vi "PlotMag.vi"(8 "error in (no error)":errorcluster, 11 "AllData In":T1 {"FlukeData"."DataAnalysisArray"."TimeStamp" format="%^<%.3X\n%x>T"; "FlukeData"."ModelDataArray"."FREQUENCY" format="%#_6f"; "FlukeData"."ModelDataArray"."TimeStamp" format="%^<%.3X\n%x>T"; "FlukeData"."PMUDataArray"."FREQUENCY" format="%#_6f"; "FlukeData"."PMUDataArray"."TimeStamp" format="%^<%.3X\n%x>T"; "NISTData"."DataAnlysisArray"."TimeStamp" format="%^<%.3X\n%x>T"; "NISTData"."DUTDataArray"."Time Stamp" format="%^<%.3X\n%x>T"; "NISTData"."NIDataArray"."Time Stamp" format="%^<%.3X\n%x>T"}) -> (0 "error out":errorcluster, 1 "NistPlot":cluster{"X":dbl, "Y":dbl}[](array[cluster]), 2 "FlukePlot":cluster{"X":dbl, "Y":dbl}[](array[cluster]))   [LabVIEW 2014]
uses:
  typedefs/Alldata.ctl
  typedefs/NISTData.ctl
  typedefs/NIDataArray.ctl
  typedefs/NIData.ctl
  typedefs/PhasorRectangular.ctl
  typedefs/DUTData.ctl
  typedefs/NICalcAnalysis.ctl
  typedefs/CalcPhasorError.ctl
  typedefs/PlotDataArrays.ctl
  typedefs/PmuRawDataCluster.ctl
  typedefs/CalcAnalysis.ctl
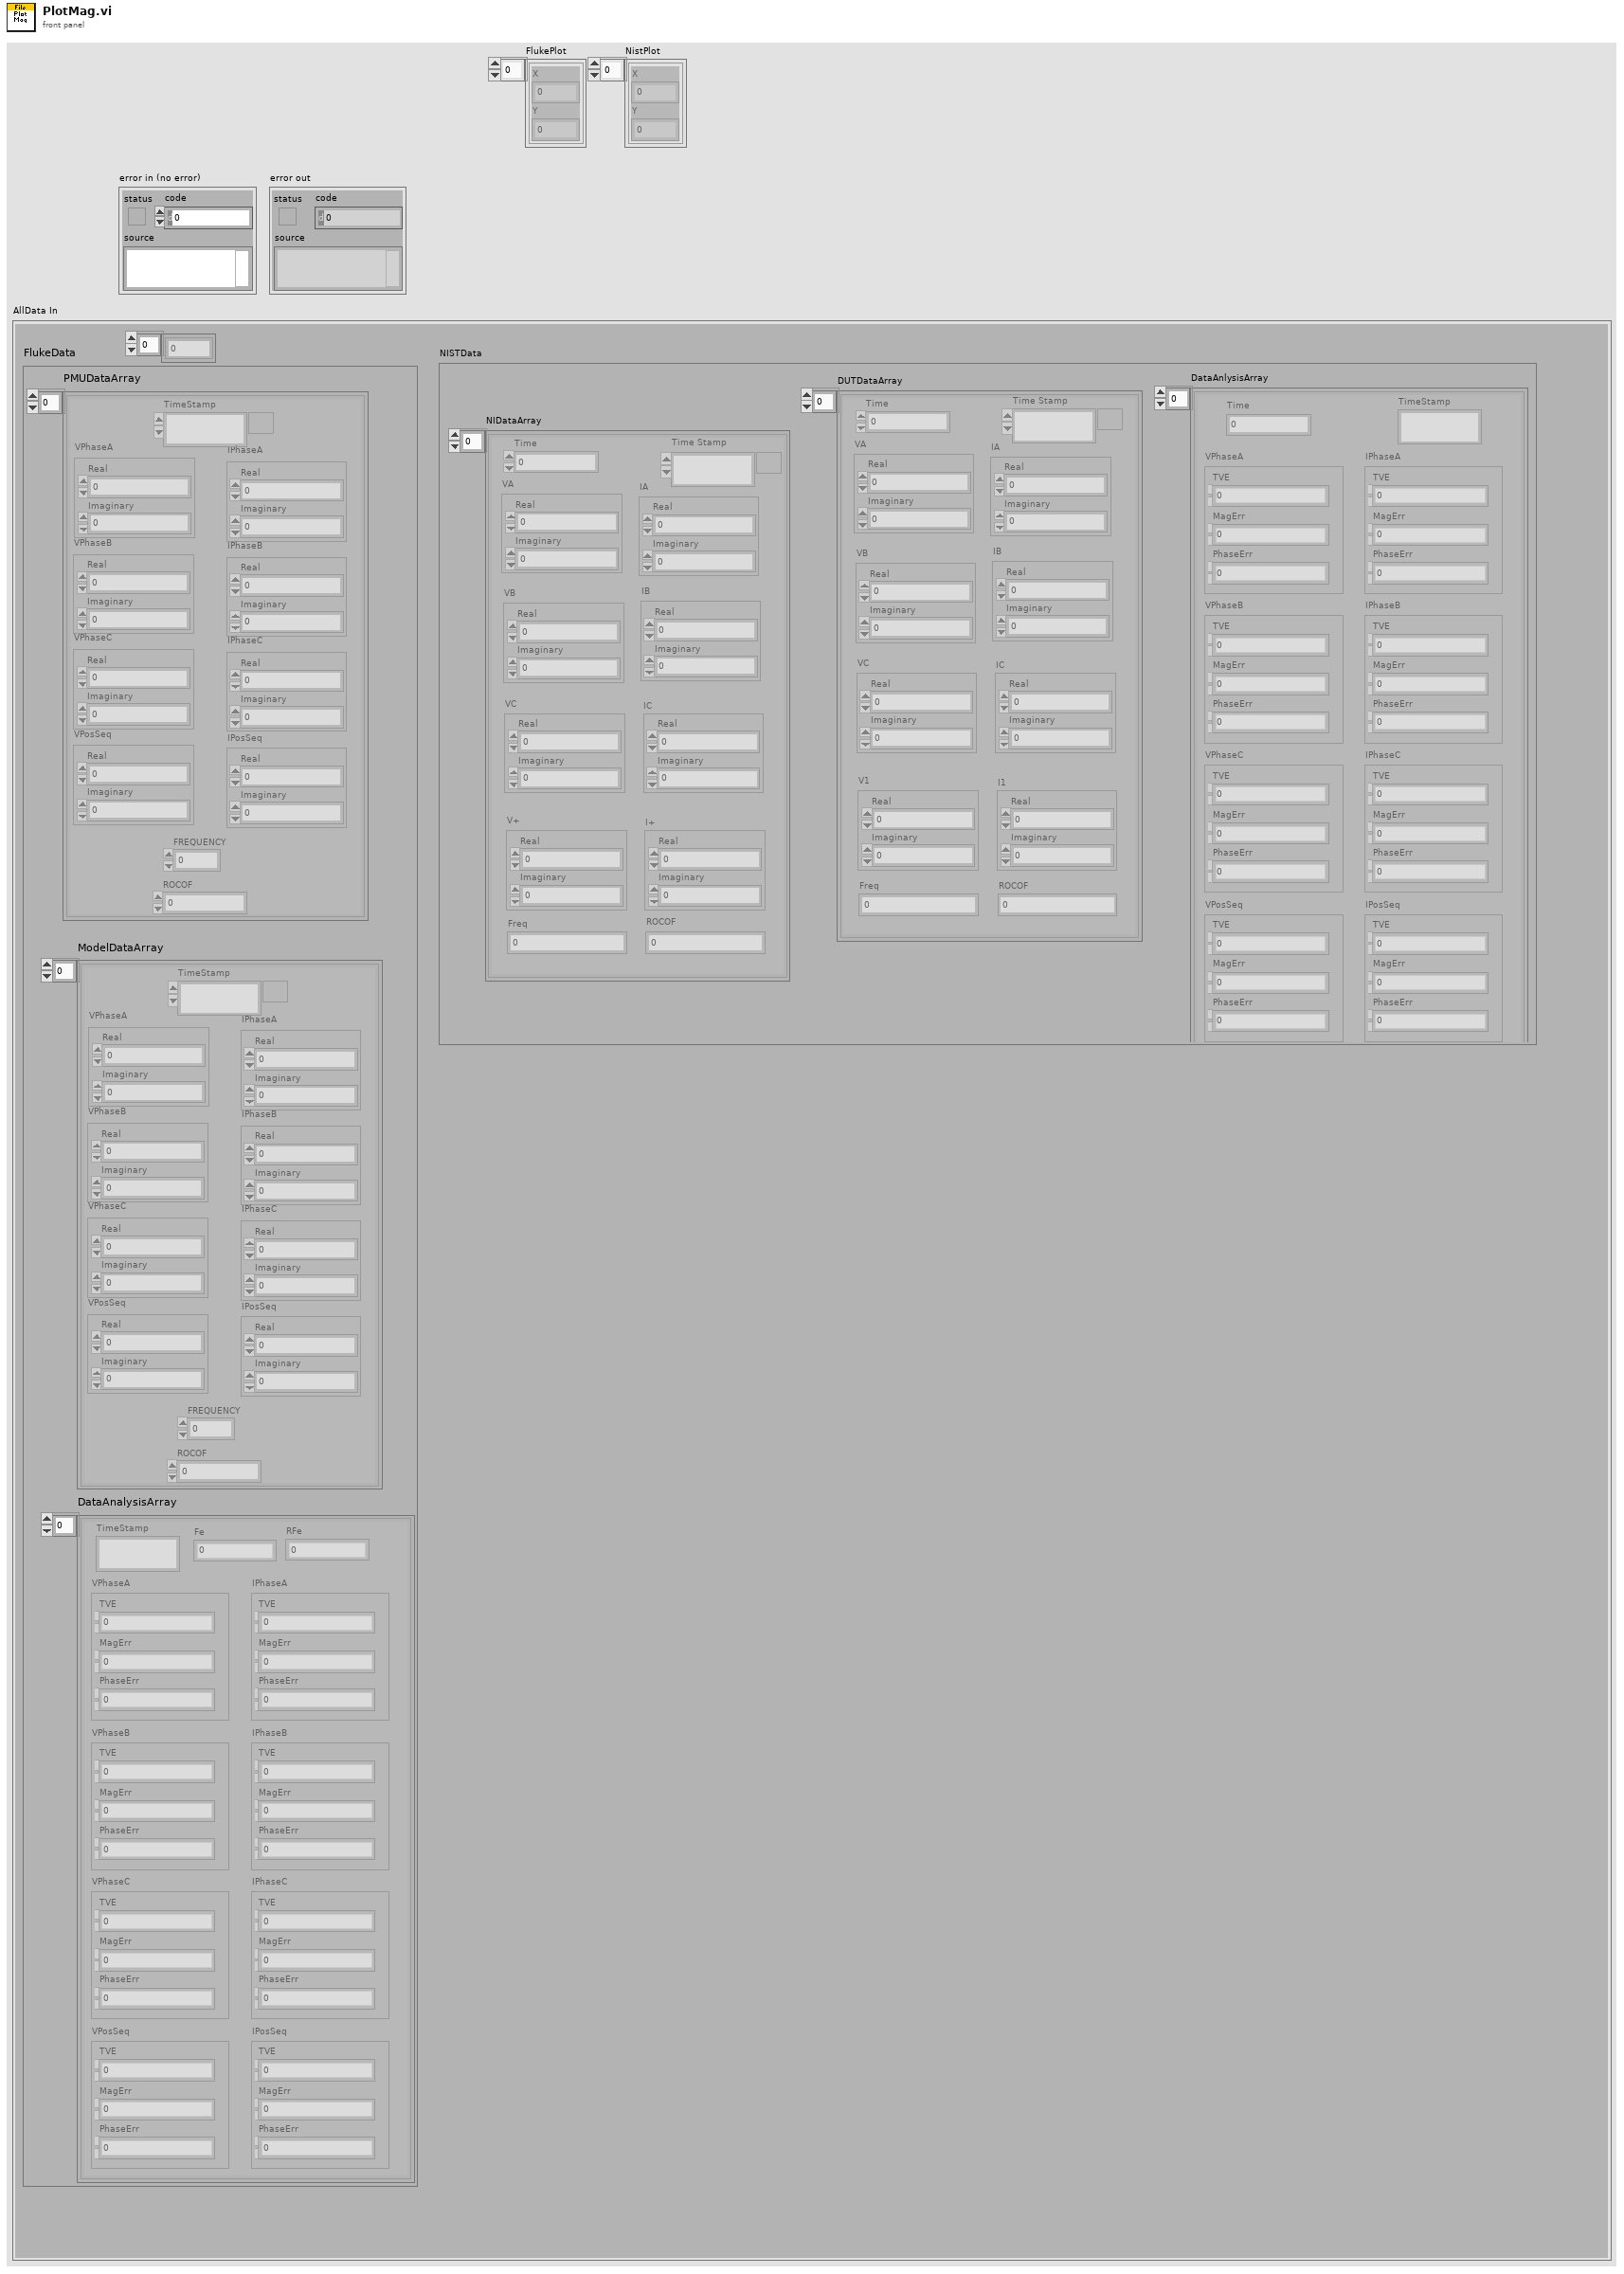
[diagram p1: front panel]
types:
  T1 = typedef "Alldata.ctl" = cluster{"NISTData":T2, "FlukeData":T9, "Params":dbl[]}
  T2 = typedef "NISTData.ctl" = cluster{"NIDataArray":T3, "DUTDataArray":T6[], "DataAnlysisArray":T7[]}
  T3 = typedef "NIDataArray.ctl" = T4[]
  T4 = typedef "NIData.ctl" = cluster{"Time":dbl, "VA":T5, "VB":T5, "VC":T5, "V+":T5, "IA":T5, "IB":T5, "IC":T5, "I+":T5, "Freq":dbl, "ROCOF":dbl, "Time Stamp":timestamp}
  T5 = typedef "PhasorRectangular.ctl" = cluster{"Real":dbl, "Imaginary":dbl}
  T6 = typedef "DUTData.ctl" = cluster{"Time":dbl, "VA":T5, "VB":T5, "VC":T5, "V1":T5, "IA":T5, "IB":T5, "IC":T5, "I1":T5, "Freq":dbl, "ROCOF":dbl, "Time Stamp":timestamp}
  T7 = typedef "NICalcAnalysis.ctl" = cluster{"Time":dbl, "VPhaseA":T8, "IPhaseA":T8, "VPhaseB":T8, "IPhaseB":T8, "VPhaseC":T8, "IPhaseC":T8, "VPosSeq":T8, "IPosSeq":T8, "Fe":dbl, "RFe":dbl, "TimeStamp":timestamp}
  T8 = typedef "CalcPhasorError.ctl" = cluster{"TVE":dbl, "MagErr":dbl, "PhaseErr":dbl}
  T9 = typedef "PlotDataArrays.ctl" = cluster{"PMUDataArray":T10[], "ModelDataArray":T10[], "DataAnalysisArray":T11[]}
  T10 = typedef "PmuRawDataCluster.ctl" = cluster{"TimeStamp":timestamp, "VPhaseA":T5, "VPhaseB":T5, "VPhaseC":T5, "VPosSeq":T5, "IPhaseA":T5, "IPhaseB":T5, "IPhaseC":T5, "IPosSeq":T5, "FREQUENCY":dbl, "ROCOF":sgl}
  T11 = typedef "CalcAnalysis.ctl" = cluster{"TimeStamp":timestamp, "VPhaseA":T8, "VPhaseB":T8, "VPhaseC":T8, "VPosSeq":T8, "IPhaseA":T8, "IPhaseB":T8, "IPhaseC":T8, "IPosSeq":T8, "Fe":dbl, "RFe":dbl}
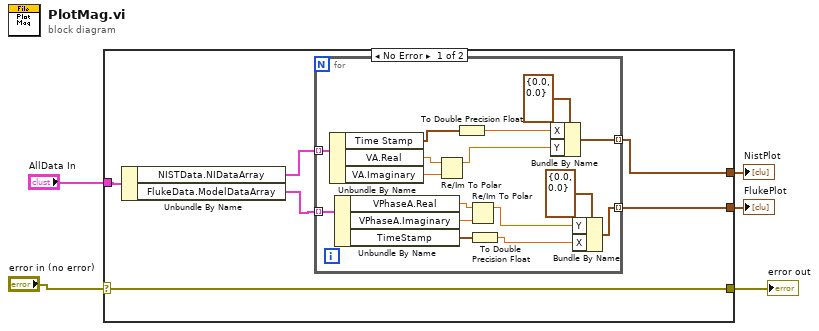
[diagram p0: block diagram]
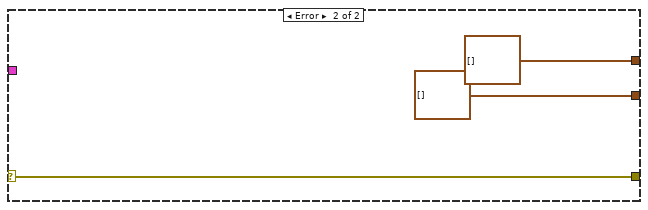
[diagram p2: hidden frame]
diagram:
  n1 = case shown="No Error" "error in (no error)" {
    selector: "error in (no error)" -> [w7 w30]
    tunnel: [w7 w30] -> w4
    tunnel: "AllData In" -> [w11 _]
    tunnel: [w6 cluster{"X":dbl, "Y":dbl}[] []] -> w1
    tunnel: [w8 cluster{"X":dbl, "Y":dbl}[] []] -> w2
    frame No Error {
      n2 = Unbundle By Name(w11) -> ("NISTData.NIDataArray"=w10:T3, "FlukeData.ModelDataArray"=w9:T10[])
      n3 = for {
        tunnel: w10 -> [w27] mode=indexing
        tunnel: w9 -> [w26] mode=indexing
        tunnel: [w17] -> w8 mode=indexing
        tunnel: [w20] -> w6 mode=indexing
        n4 = Unbundle By Name(w27) -> ("Time Stamp"=w22:timestamp, "VA.Real"=w13:dbl, "VA.Imaginary"=w14:dbl)
        n5 = Unbundle By Name(w26) -> ("VPhaseA.Real"=w24:dbl, "VPhaseA.Imaginary"=w25:dbl, "TimeStamp"=w19:timestamp)
        n6 = Re/Im To Polar(2:w14, 3:w13) -> (1:w12:dbl)  [unwired: 1 out]
        n7 = To Double Precision Float(number=w22) -> (double precision float=w21:dbl)
        n8 = Re/Im To Polar(2:w25, 3:w24) -> (1:w15:dbl)  [unwired: 1 out]
        n9 = To Double Precision Float(number=w19) -> (double precision float=w16:dbl)
        n10 = Bundle By Name(cluster=cluster{"X":dbl, "Y":dbl} {"X"=0.0, "Y"=0.0} ("input cluster"), "X"=w21, "Y"=w12) -> (w20:cluster{"X":dbl, "Y":dbl})
        n11 = Bundle By Name(cluster=cluster{"X":dbl, "Y":dbl} {"X"=0.0, "Y"=0.0} ("input cluster"), "Y"=w15, "X"=w16) -> (w17:cluster{"X":dbl, "Y":dbl})
      }
    }
    frame Error {
    }
  }
  "error out" <- w4
  "FlukePlot" <- w2
  "NistPlot" <- w1
